vi "定时.vi"(11 "初始化":bool) -> (2 "时间":dbl)   [LabVIEW 2011]
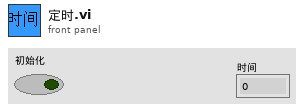
[diagram p1: front panel]
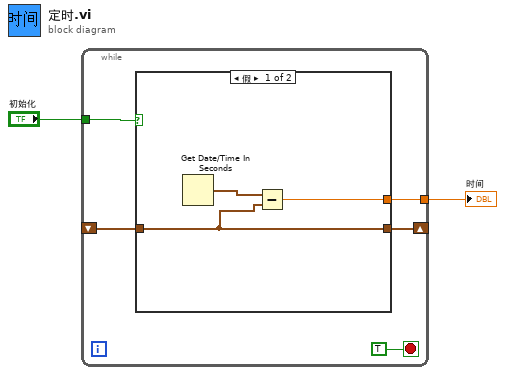
[diagram p0: block diagram]
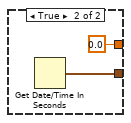
[diagram p2: hidden frame]
diagram:
  n1 = while {
    tunnel: "初始化" -> [w6]
    shift-right: [w4] -> _
    shift-left: _ -> [w5]
    tunnel: [w3] -> w1
    stop <- TRUE stop-if-true
    n2 = case shown="假" w6 {
      tunnel: w5 -> [w9 _]
      tunnel: [w9 w12] -> w4
      tunnel: [w8 0.0] -> w3
      frame False {
        n3 = Get Date/Time In Seconds() -> (seconds since 1Jan1904=w10:timestamp)
        n4 = Subtract(x=w10, y=w9) -> (x-y=w8:dbl)
      }
      frame True {
        n5 = Get Date/Time In Seconds() -> (seconds since 1Jan1904=w12:timestamp)
      }
    }
  }
  "时间" <- w1
